vi "get_soft_limit_XYZ.vi"(8 "error in (no error)":errorcluster caption="错误输入（无错误）", 11 "MotorSystem 输入":refnum<class "MotorSystem.lvclass">) -> (0 "error out":errorcluster caption="错误输出", 2 "soft limit":T1={"X"={"min"=-12.0, "max"=12.0}, "Y"={"min"=-12.0, "max"=12.0}, "Z"={"min"=0.0, "max"=350.0}}, 3 "MotorSystem 输出":refnum<class "MotorSystem.lvclass">)   [LabVIEW 2016, in "MotionControl_UFO_3DOF.lvlib" / "MotorSystem.lvclass"]
uses:
  <userlib>/MotionControl_UFO_3DOF/MotorSystem/MotorSystem.lvclass
  <userlib>/MotionControl_UFO_3DOF/MotorSystem/MotorSystem.lvclass/MotorSystem.ctl
  <userlib>/MotionControl_UFO_3DOF/OneMotion/OneMotion.lvclass/OneMotion.ctl
  <userlib>/MotionControl_UFO_3DOF/OneMotion/OneMotion.lvclass
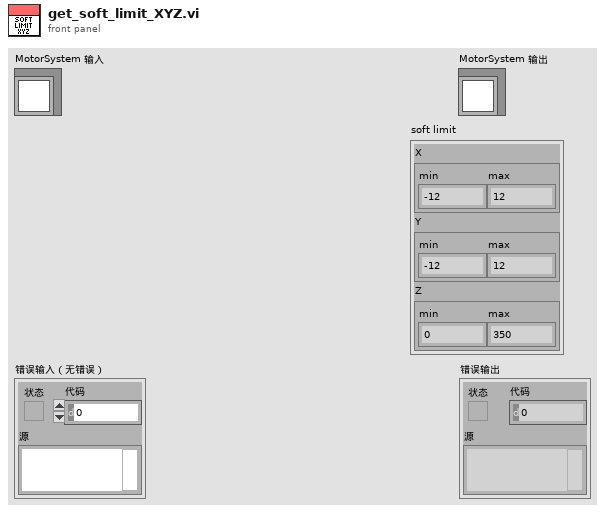
[diagram p1: front panel]
types:
  T1 = cluster{"X":cluster{"min":dbl, "max":dbl}, "Y":cluster{"min":dbl, "max":dbl}, "Z":cluster{"min":dbl, "max":dbl}}
  T2 = typedef "MotionControl_UFO_3DOF.lvlib/MotorSystem.lvclass/MotionCluster.ctl" = cluster{"OneMotion.lvclass":refnum<class "OneMotion.lvclass">, "connected?":bool, "default enabled?":bool, "enabled?":bool}
  T3 = cluster{"[0]":cluster{"min":dbl, "max":dbl}, "[1]":cluster{"min":dbl, "max":dbl}, "[2]":cluster{"min":dbl, "max":dbl}}
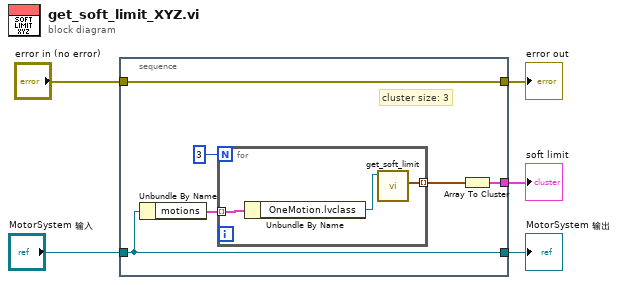
[diagram p0: block diagram]
diagram:
  n1 = stacked-sequence {
    tunnel: [w11] -> w5
    tunnel: [w9] -> w3
    tunnel: "MotorSystem 输入" -> [w9]
    tunnel: "error in (no error)" -> [w11]
    tunnel: [w6] -> w1
    frame #0 {
      # "cluster size: 3"
      n2 = Unbundle By Name(w9) -> ("motions"=w8:T2[])
      n3 = for {
        N: 3 -> [_]
        tunnel: w8 -> [w14] mode=indexing
        tunnel: [w12] -> w7 mode=indexing
        n4 = Unbundle By Name(w14) -> ("OneMotion.lvclass"=w13:refnum<class "OneMotion.lvclass">)
        n5 = call <userlib>:"get_soft_limit.vi"("OneMotion输入"=w13) -> ("soft limit"=w12:cluster{"min":dbl, "max":dbl})  [unwired: 8 in, 2 out]
      }
      n6 = Array To Cluster(array=w7) -> (cluster=w6:T3)
    }
  }
  "error out" <- w5
  "MotorSystem 输出" <- w3
  "soft limit" <- w1
